vi "Show Python UI.vi"(7 "Server Alias":string, 8 "error in (no error)":errorcluster) -> (0 "error out":errorcluster)   [LabVIEW 2013, in "TS.lvlib"]
doc: "This is likely unnecessary most of the time. There is a tkinter GUI available on the Python side for information and debugging purposes. This VI will show that GUI."
uses:
  TS.lvlib
  LabVIEW Python Connector Message.ctl
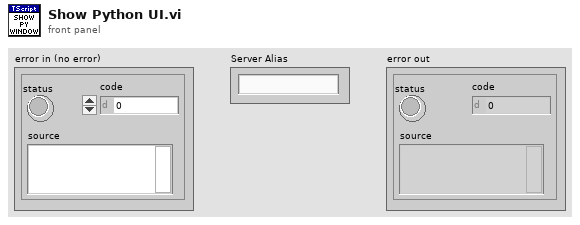
[diagram p1: front panel]
types:
  T1 = typedef "TS.lvlib/LabVIEW Python Connector Message.ctl" = cluster{"Command":string, "Data":string[], "Script ID":i64, "LabVIEW Server ID":string, "Python Message ID":i32}
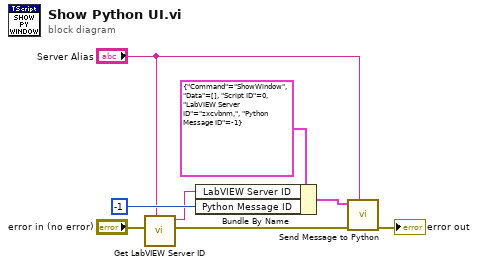
[diagram p0: block diagram]
diagram:
  n1 = call "Get LabVIEW Server ID.vi"("Server Alias"="Server Alias", "Error In"="error in (no error)") -> ("Error Out"=w3:errorcluster, "LabVIEW Server ID"=w2:string)  [unwired: 8 in]
  n2 = Bundle By Name(cluster=T1 {"Command"="ShowWindow", "Data"=[], "Script ID"=0, "LabVIEW Server ID"="zxcvbnm,", "Python Message ID"=-1} ("Message"), "LabVIEW Server ID"=w2, "Python Message ID"=-1) -> (w6:T1)
  n3 = call "Send Message to Python.vi"("Server Alias"="Server Alias", "error in (no error)"=w3, "Message"=w6) -> ("error out"=→"error out":errorcluster)  [unwired: 8 in]
